vi "Start Server.vi"(10 "remote port":u16=8080) -> ()   [LabVIEW 2009]
doc: "This VI starts the XML-RPC server in a new thread (non-blocking)"
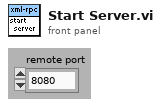
[diagram p1: front panel]
types:
  T1 = enum32{"invalid app kind", "Development System", "Run Time System", "Student Edition", "Embedded LabVIEW", "Evaluation", "Custom"}
  T2 = enum32{"Bad", "Idle", "Run top level", "Running"}
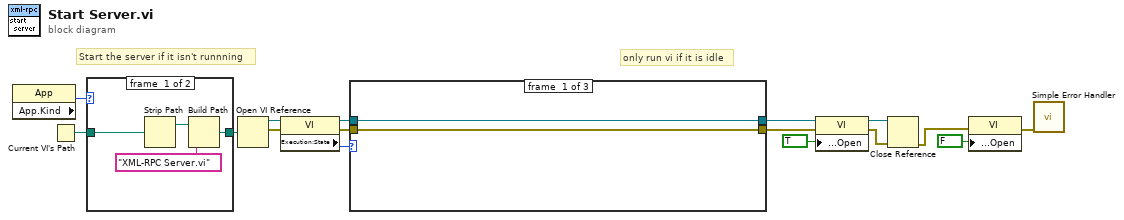
[diagram p0: block diagram]
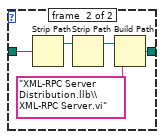
[diagram p2: hidden frame]
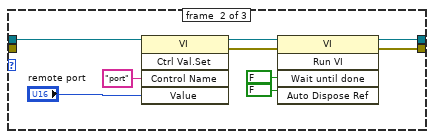
[diagram p3: hidden frame]
diagram:
  # "Start the server if it isn't runnning"
  # "only run vi if it is idle"
  n1 = property class="App"() -> ("App.Kind"=w9:T1)  [unwired: 2 in, 2 out]
  n2 = Current VI's Path() -> (path=w11:path)
  n3 = case shown="Default" w9 {
    tunnel: w11 -> [w20 w25]
    tunnel: [w18 w24] -> w10
    frame #0 {
      n4 = Strip Path(path=w20) -> (stripped path=w19:path)  [unwired: 1 out]
      n5 = Build Path(base path=w19, name or relative path="XML-RPC Server.vi") -> (appended path=w18:path)
    }
    frame #1 {
      n6 = Strip Path(path=w25) -> (stripped path=w23:path)  [unwired: 1 out]
      n7 = Strip Path(path=w23) -> (stripped path=w22:path)  [unwired: 1 out]
      n8 = Build Path(base path=w22, name or relative path="XML-RPC Server Distribution.llb\\XML-RPC Server.vi") -> (appended path=w24:path)
    }
  }
  n9 = Open VI Reference(vi path=w10) -> (vi reference=w12:refnum<vi>, error out=w13:errorcluster)  [unwired: 5 in]
  n10 = property class="VI"(reference=w12, error in=w13) -> (reference out=w15:refnum<vi>, error out=w14:errorcluster, "Execution:State"=w16:T2)
  n11 = case shown="\"Idle\"" w16 {
    tunnel: [w27 w35 w38] -> w7
    tunnel: w15 -> [w27 w32 w38]
    tunnel: w14 -> [w26 _ w37]
    tunnel: [w26 w33 w37] -> w4
    frame #0 {
    }
    frame #1 {
      n12 = invoke class="VI" method="Ctrl Val.Set"(reference=w32, "Control Name"="port", "Value"="remote port") -> (reference out=w31:refnum<vi>, error out=w30:errorcluster)  [unwired: 2 in, 3 out]
      n13 = invoke class="VI" method="Run VI"(reference=w31, error in=w30, "Wait until done"=FALSE, "Auto Dispose Ref"=FALSE ("Auto Dispose Reference")) -> (reference out=w35:refnum<vi>, error out=w33:errorcluster)  [unwired: 1 in, 3 out]
    }
    frame #2 {
    }
  }
  n14 = property class="VI"(reference=w7, error in=w4, "Front Panel.Open"=TRUE ("Front Panel Window:Open")) -> (reference out=w5:refnum<vi>, error out=w6:errorcluster)
  n15 = Close Reference(reference=w5, error in (no error)=w6) -> (error out=w3:errorcluster)
  n16 = property class="VI"(error in=w3, "Front Panel.Open"=FALSE ("Front Panel Window:Open")) -> (error out=w1:errorcluster)  [unwired: 1 in, 1 out]
  n17 = call <vilib>:"Simple Error Handler.vi"("error in (no error)"=w1) -> ()  [unwired: 4 in, 5 out]
